vi "smtp_email.vi"(8 "error in (no error)":errorcluster, 10 "subject":string, 11 "plain text message":string) -> (0 "error out":errorcluster, 2 "invalid recipients":string[](array[string]))   [LabVIEW 2019]
uses:
  <vilib>/smtpClient/Set Message Text.vi
  <vilib>/smtpClient/LabVIEWSMTPClient.lvlib
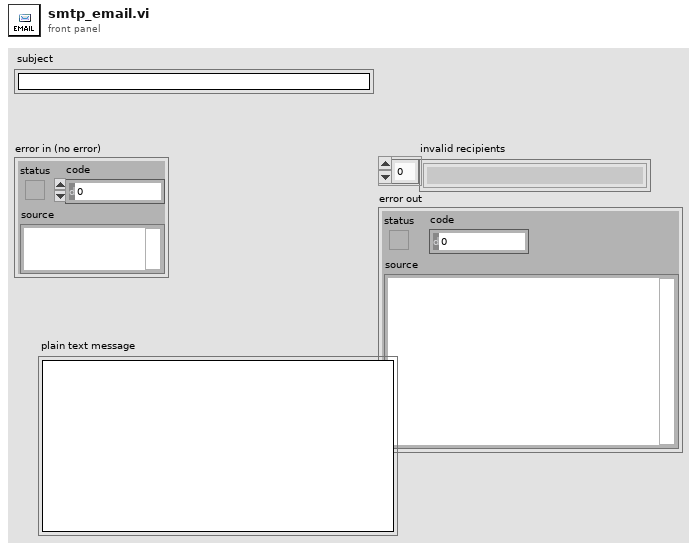
[diagram p1: front panel]
types:
  T1 = typedef "LabVIEWSMTPClient.lvlib/SmtpClientHandle.ctl" = refnum<k1>
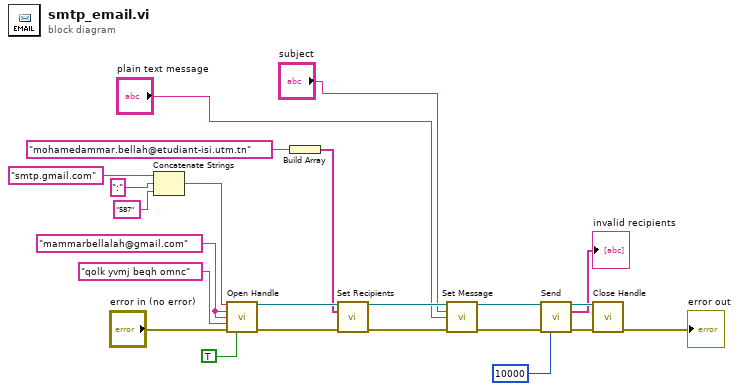
[diagram p0: block diagram]
diagram:
  w13 = "mammarbellalah@gmail.com" ("from")
  n1 = Concatenate Strings("smtp.gmail.com" ("string"), ":" ("string"), "587" ("string")) -> (w14:string)
  n2 = call <vilib>:"Open Handle.vi"("server address"=w14, "from"=w13, "username"=w13, "password"="qolk yvmj beqh omnc", "error in (no error)"="error in (no error)", "use TLS (false)"=TRUE) -> ("handle out"=w23:T1, "error out"=w20:errorcluster)  [unwired: 8 in]
  n3 = Build Array("mohamedammar.bellah@etudiant-isi.utm.tn") -> (w9:string[])
  n4 = call <vilib>:"Set Recipients.vi"("handle in"=w23, "to"=w9, "error in (no error)"=w20) -> ("handle out"=w22:T1, "error out"=w19:errorcluster)  [unwired: 11 in]
  n5 = call-poly <vilib>:"Set Message.vi"("handle in"=w22, "subject"="subject", "plain text message"="plain text message", "error in (no error)"=w19) -> ("handle out"=w6:T1, "error out"=w5:errorcluster)  [unwired: 10 in]
  n6 = call <vilib>:"Send.vi"("handle in"=w6, "error in (no error)"=w5, "timeout in ms (10000)"=10000) -> ("handle out"=w21:T1, "invalid recipients"=→"invalid recipients":string[], "error out"=w18:errorcluster)  [unwired: 10 in]
  n7 = call <vilib>:"Close Handle.vi"("handle in"=w21, "error in (no error)"=w18) -> ("error out"=→"error out":errorcluster)  [unwired: 12 in, 1 out]
